vi "AdaFruit.vi"(0 "Blink Rate":u32, 1 "Number of Lights":u8, 2 "Gear In?":bool) -> ()   [LabVIEW 2016]
doc: "ADXL362 SPI Accelerometer\n\nThis example shows how to use the Analog Devices ADXL362 Accelerometer sensor connected to SPI.\n\nThis example expects a USB cable connected from your development PC to the Type B USB Jack (next to the power input) on the roboRIO."
uses:
  <vilib>/Rock Robotics/SystemInterfaces/spilib/spi_bus.ctl
  <vilib>/Rock Robotics/WPI/SPI/WPI_SPIMode.ctl
panel:
  in  "Global Max\nBrightness":u8(slide)=4 max=31 scale=0.0..31.0
  out "ONOFF":bool
  in  "Blinky End":u8
  in  "Chip Select Active High (F)":bool
  in  "Mode (3)":T1=enum."Mode 3 (Clk Idle High,Sample on Trailing)"
  in  "Clock Rate (Hz)":dbl=500000.0
  in  "error in":errorcluster
  in  "SPI Bus":T2=enum."SPI On-Board, CS1"
  out "error out":errorcluster
  in  "stop":bool
  # "Set these inputs before running."
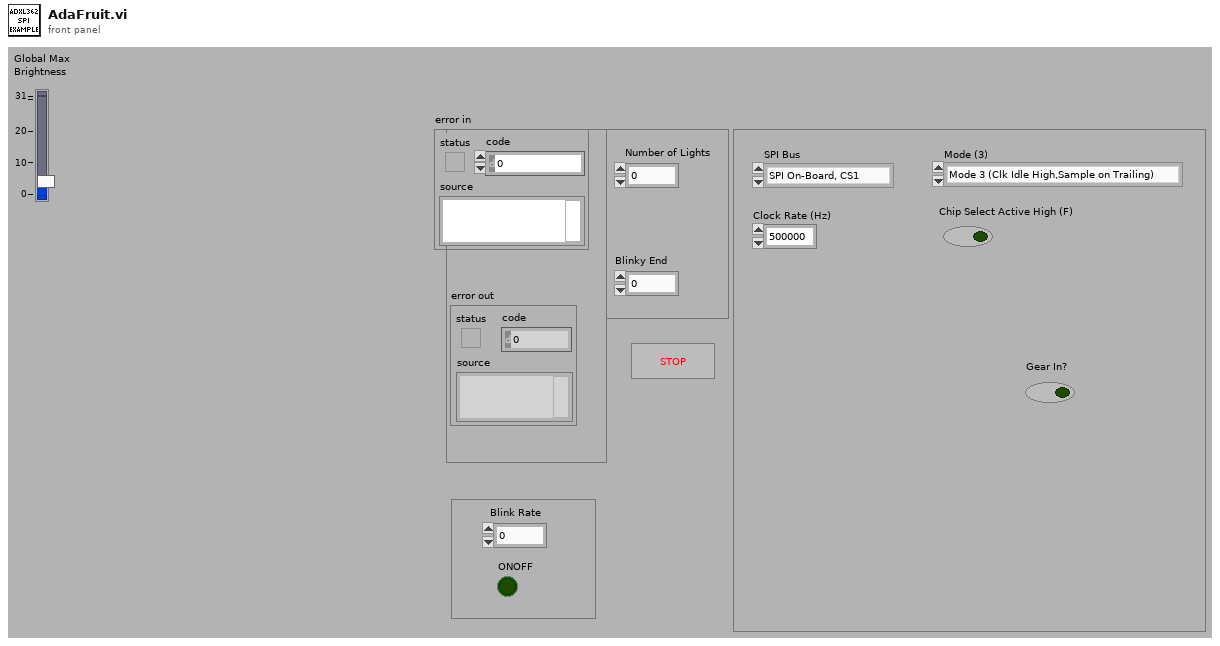
[diagram p1: front panel]
types:
  T1 = typedef "WPI_SPIMode.ctl" = enum16{"Mode 0 (Clk Idle Low,Sample on Leading)", "Mode 1 (Clk Idle Low,Sample on Trailing)", "Mode 2 (Clk Idle High,Sample on Leading)", "Mode 3 (Clk Idle High,Sample on Trailing)"}
  T2 = typedef "spi_bus.ctl" = enum16{"SPI On-Board, CS0", "SPI On-Board, CS1", "SPI On-Board, CS2", "SPI On-Board, CS3", "SPI MXP", "Invalid"}
  T3 = typedef "WPI_SPIDevRef.ctl" = cluster{"DevStatus":errorcluster, "Handle":i32, "SPI Bus":T2}
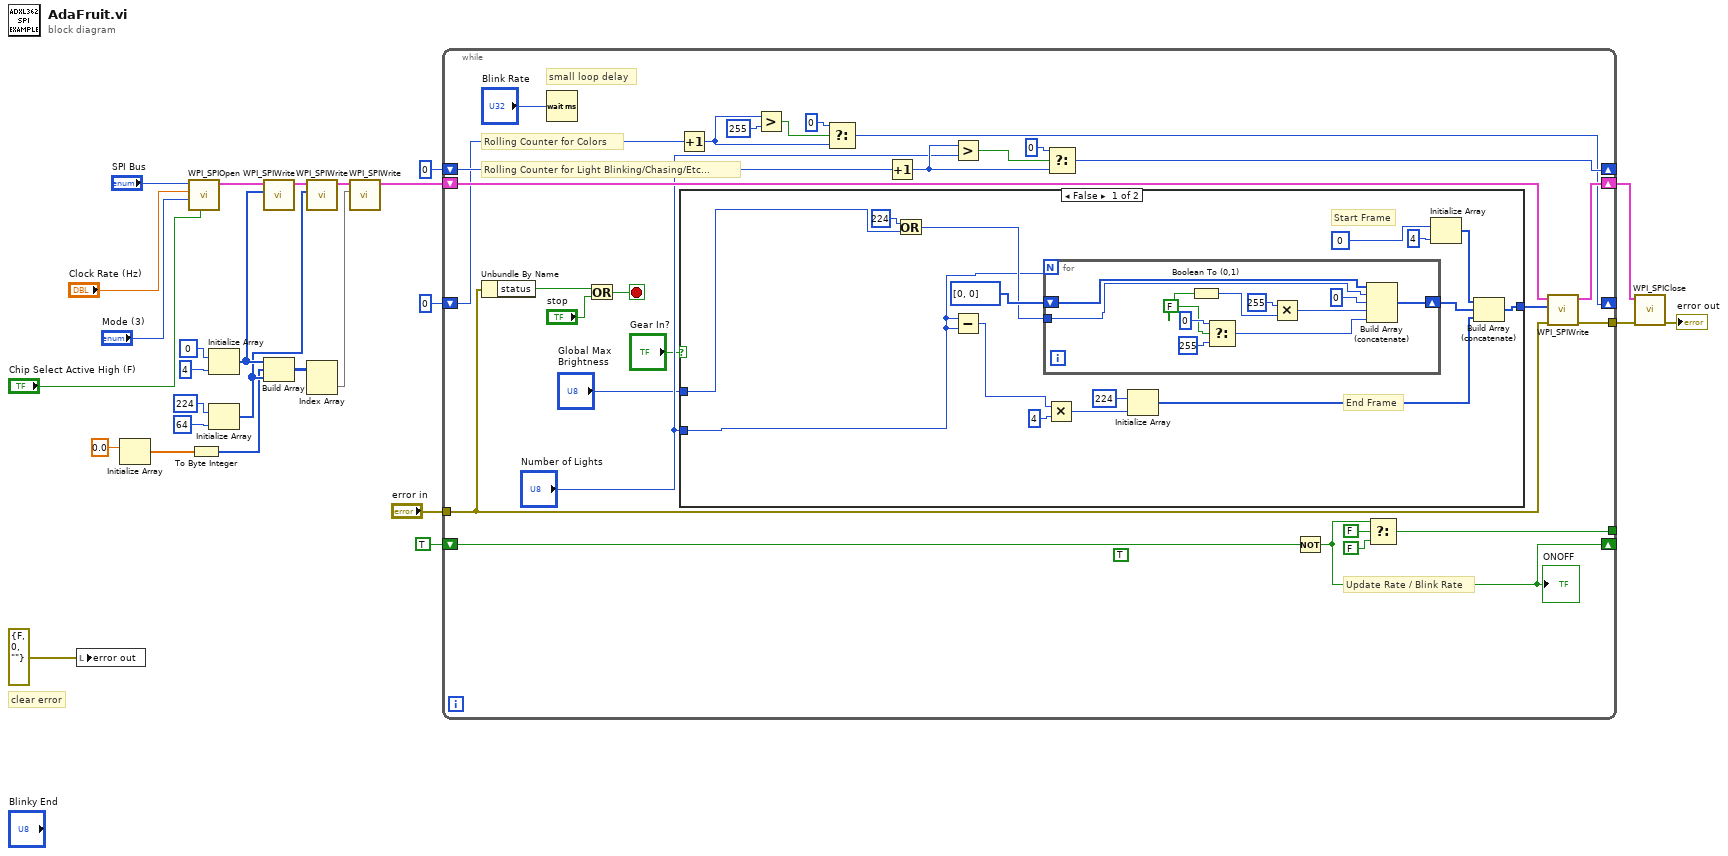
[diagram p0: block diagram]
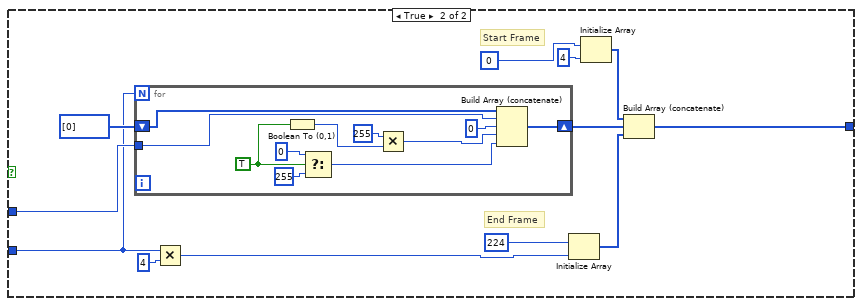
[diagram p2: hidden frame]
diagram:
  # "clear error"
  n1 = local write "error out"(errorcluster {"status"=FALSE, "code"=0, "source"=""} ("error out")) -> ()
  n2 = Initialize Array(0.0 ("element")) -> (w4:dbl[])  [unwired: 1 in]
  n3 = call <vilib>:"WPI_SPIOpen.vi"("Chip Select Active High (F)"="Chip Select Active High (F)", "Mode (3)"="Mode (3)", "Clock Rate (Hz)"="Clock Rate (Hz)", "SPI Bus"="SPI Bus") -> ("SPIDevRef"=w17:T3)  [unwired: 6 in, 1 out]
  n4 = To Byte Integer(number=w4) -> (8bit integer=w3:i8[])
  n5 = Initialize Array(u8 0 ("Data To Send"), u8 4 ("dimension size")) -> (w9:u8[])
  n6 = Initialize Array(u8 224 ("Data To Send"), u8 64 ("dimension size")) -> (w8:u8[])
  n7 = call <vilib>:"WPI_SPIWrite.vi"("Data To Send"=w9, "SPIDevRef"=w17) -> ("SPIDevRef"=w13:T3)  [unwired: 7 in, 2 out]
  n8 = Build Array(w9, w3, w8) -> (w2:u8[][])
  n9 = call <vilib>:"WPI_SPIWrite.vi"("Data To Send"=w8, "SPIDevRef"=w13) -> ("SPIDevRef"=w6:T3)  [unwired: 7 in, 2 out]
  n10 = Index Array(array=w2) -> (element=w1:u8[])  [unwired: 2 in]
  n11 = call <vilib>:"WPI_SPIWrite.vi"("Data To Send"=w1, "SPIDevRef"=w6) -> ("SPIDevRef"=w7:T3)  [unwired: 7 in, 2 out]
  n12 = while {
    shift-right: [w54] -> w24
    shift-left: w7 -> [w52]
    tunnel: "error in" -> [w50]
    tunnel: [w53] -> w14
    tunnel: [w45] -> _
    shift-right: [w43] -> _
    shift-left: TRUE -> [w44]
    shift-right: [w39] -> _
    shift-left: 0 -> [w38]
    shift-right: [w34] -> _
    shift-left: 0 -> [w32]
    stop <- w49 stop-if-true
    (unwired) TRUE
    # "Update Rate / Blink Rate"
    # "Rolling Counter for Light Blinking/Chasing/Etc..."
    # "Rolling Counter for Colors"
    # "small loop delay"
    n13 = Unbundle By Name(w50) -> ("status"=w51:bool)
    n14 = Wait (ms)(milliseconds to wait="Blink Rate") -> ()  [unwired: 1 out]
    n15 = Or(x=w51, y="stop") -> (x .or. y?=w49:bool)
    n16 = Increment(x=w32) -> (x+1=w35:u8)
    n17 = case shown="False" "Gear In?" {
      tunnel: "Number of Lights" -> [w56 w86]
      tunnel: [w58 w83] -> w29
      tunnel: "Global Max\nBrightness" -> [w57 w93]
      frame False {
        # "End Frame"
        # "Start Frame"
        n18 = Or(x=u8 224, y=w57) -> (x .or. y?=w60:u8)
        n19 = Subtract(x=w56, y=w56) -> (x-y=w64:u8)
        n20 = for {
          N: w56 -> [_]
          tunnel: w60 -> [w77]
          shift-right: [w73] -> w69
          shift-left: i16[] [0, 0] -> [w72]
          w71 = FALSE
          n21 = Boolean To (0,1)(Boolean=w71) -> (0, 1=w80:i16)
          n22 = Select(t=u8 0, s=w71, f=u8 255) -> (s? t:f=w74:u8)
          n23 = Multiply(x=u8 255, y=w80) -> (x*y=w75:i16)
          n24 = Build Array (concatenate)(w72, w77, u8 0 ("element"), w75, w74) -> (w73:i16[])
        }
        n25 = Multiply(x=w64, y=4) -> (x*y=w66:i32)
        n26 = Initialize Array(u8 224 ("Data To Send"), w66) -> (w68:u8[])
        n27 = Initialize Array(u8 0 ("Data To Send"), u8 4 ("dimension size")) -> (w67:u8[])
        n28 = Build Array (concatenate)(w67, w69, w68) -> (w58:i16[])
      }
      frame True {
        # "End Frame"
        # "Start Frame"
        n29 = for {
          N: w86 -> [_]
          tunnel: w93 -> [w99]
          shift-right: [w95] -> w87
          shift-left: i16[] [0] -> [w94]
          w100 = TRUE
          n30 = Boolean To (0,1)(Boolean=w100) -> (0, 1=w103:i16)
          n31 = Select(t=u8 0, s=w100, f=u8 255) -> (s? t:f=w96:u8)
          n32 = Multiply(x=u8 255, y=w103) -> (x*y=w97:i16)
          n33 = Build Array (concatenate)(w94, w99, u8 0 ("element"), w97, w96) -> (w95:i16[])
        }
        n34 = Multiply(x=w86, y=4) -> (x*y=w88:i32)
        n35 = Initialize Array(u8 224 ("Data To Send"), w88) -> (w85:u8[])
        n36 = Initialize Array(u8 0 ("Data To Send"), u8 4 ("dimension size")) -> (w84:u8[])
        n37 = Build Array (concatenate)(w84, w87, w85) -> (w83:i16[])
      }
    }
    n38 = Greater?(x=w35, y=255) -> (0:w36:bool)
    n39 = Select(t=0, s=w36, f=w35) -> (s? t:f=w34:i32)
    n40 = Increment(x=w38) -> (x+1=w40:u8)
    n41 = Greater?(x=w40, y="Number of Lights") -> (0:w41:bool)
    n42 = Select(t=0, s=w41, f=w40) -> (s? t:f=w39:i32)
    n43 = Not(x=w44) -> (.not. x?=w43:bool)
    "ONOFF" <- w43
    n44 = Select(t=w43, s=FALSE, f=FALSE) -> (s? t:f=w45:bool)
    n45 = call <vilib>:"WPI_SPIWrite.vi"("error in (no error)"=w50, "Data To Send"=w29, "SPIDevRef"=w52) -> ("error out"=w53:errorcluster, "SPIDevRef"=w54:T3)  [unwired: 6 in, 1 out]
  }
  n46 = call <vilib>:"WPI_SPIClose.vi"("error in (no error)"=w14, "SPIDevRef"=w24) -> ("error out"=→"error out":errorcluster)  [unwired: 9 in]
